vi "TableSandbox.vi"() -> ()   [LabVIEW 2013]
uses:
  <vilib>/Utility/miscctls.llb/LVRowAndColumnTypeDef.ctl
  <vilib>/Utility/miscctls.llb/LVBoundsTypeDef.ctl
  <vilib>/Utility/miscctls.llb/LVFontTypeDef.ctl
  <vilib>/Utility/miscctls.llb/LVPositionTypeDef.ctl
  <vilib>/Utility/miscctls.llb/LVRowAndColumnUnsignedTypeDef.ctl
  <vilib>/event_ctls.llb/eventsource.ctl
  <vilib>/event_ctls.llb/lveventtype.ctl
  <vilib>/Utility/miscctls.llb/LVPoint32TypeDef.ctl
  <vilib>/event_ctls.llb/eventvkey.ctl
  <vilib>/Utility/cursorutil.llb/Set Cursor (Icon Pict).vi
panel:
  out "Mouse\nUp":bool
  out "Mouse\nDown":bool
  out "data cols":i32
  out "data rows":i32
  in  "Enable diagnostics?":bool
  out "Active Cell:Cell Size":T1
  out "Color Box 3":u32(colorbox)
  out "Invoke: Point to Row-Column":cluster{"Cell Position":T2, "In Bounds?":bool}
  out "Active Cell:Position":T3
  out "Color Box 2":u32(colorbox)
  out "Active Cell:Cell Justification":enum16{"Left", "Center", "Right"}(ring)
  out "Active Cell:Cell Font":T4
  out "Active Cell:Cell Background Color":u32
  out "Active Cell:Active Cell":T2
  out "Row Header \nStrings[]":string[](array[string])
  out "Number of Rows":u32
  out "Number of Columns":u32
  out "Index Values":T5
  out "Edit Position":T2
  out "Content Rect\nPosition":T3
  out "Content Rect\nBounds":T1
  out "Size":T1
  out "Column Header \nStrings[]":string[](array[string])
  out "Autosizing Row Height":bool
  out "Visible Items:Vertical Scrollbar Visible":bool
  out "Visible Items:Vertical Lines Visible":bool
  out "Visible Items:Row Headers Visible":bool
  out "Visible Items:Index Visible":bool
  out "Visible Items:Horizontal Scrollbar Visible":bool
  out "Visible Items:Horizontal Lines Visible":bool
  out "Visible Items:Column Headers Visible":bool
  out "Smooth Horizontal Scrolling":bool
  out "Color Box":u32(colorbox)
  out "Selection Start":T2
  out "Selection Size":T2
  out "Selection Color":u32
  in  "Mode Col":i32=5
  in  "Tab Control":enum32{"Mouse Events", "Keyboard events"}(tab)
  out "Mouse Move\nIn Bounds?":bool
  out "Mouse Move\nCell Position":T2
  out "Mouse Move":T9={"Source"=0, "Type"=enum."Value Change", "Time"=0, "CtlRef"=refnum, "Coords"={"Horizontal"=0, "Vertical"=0}} {"Source" items=["LabVIEW UI"=0, "ActiveX"=1, "User Event"=25]}
  out "Mouse Leave":T10={"Source"=0, "Type"=enum."Value Change", "Time"=0, "CtlRef"=refnum} {"Source" items=["LabVIEW UI"=0, "ActiveX"=1, "User Event"=25]}
  out "Mouse Enter":T10={"Source"=0, "Type"=enum."Value Change", "Time"=0, "CtlRef"=refnum} {"Source" items=["LabVIEW UI"=0, "ActiveX"=1, "User Event"=25]}
  out "Mouse Up Event":T11={"Source"=0, "Type"=enum."Value Change", "Time"=0, "CtlRef"=refnum, "Coords"={"Horizontal"=0, "Vertical"=0}, "Button"=0, "Mods"={"Double Click"=FALSE, "Menu Key"=FALSE}, "PlatMods"={"Shift"=FALSE, "Ctrl"=FALSE, "Alt"=FALSE, "Cmd"=FALSE, "Opt"=FALSE}, "Invoke: Coords to row-col"={"In Bounds?"=FALSE, "Cell Position"={"Row"=0, "Column"=0}}} {"Source" items=["LabVIEW UI"=0, "ActiveX"=1, "User Event"=25]}
  out "down within digitals?":bool
  out "Shortcut Menu Activation? Event":T12={"Source"=0, "Type"=enum."Value Change", "Time"=0, "CtlRef"=refnum, "MenuRef"=refnum, "Coords"={"Horizontal"=0, "Vertical"=0}, "SubObj"=refnum, "Invoke: Coords to row-col"={"In Bounds?"=FALSE, "Cell Position"={"Row"=0, "Column"=0}}} {"Source" items=["LabVIEW UI"=0, "ActiveX"=1, "User Event"=25]}
  out "Mouse Down Event":T11={"Source"=0, "Type"=enum."Value Change", "Time"=0, "CtlRef"=refnum, "Coords"={"Horizontal"=0, "Vertical"=0}, "Button"=0, "Mods"={"Double Click"=FALSE, "Menu Key"=FALSE}, "PlatMods"={"Shift"=FALSE, "Ctrl"=FALSE, "Alt"=FALSE, "Cmd"=FALSE, "Opt"=FALSE}, "Invoke: Coords to row-col"={"In Bounds?"=FALSE, "Cell Position"={"Row"=0, "Column"=0}}} {"Source" items=["LabVIEW UI"=0, "ActiveX"=1, "User Event"=25]}
  out "down within edit":bool
  out "Button \n(Mouse Down?)":u16
  out "Key Down Event":T14={"Source"=0, "Type"=enum."Value Change", "Time"=0, "CtlRef"=refnum, "Char"=0, "VKey"=enum."ASCII", "ScanCode"=0, "Mods"={"Num Pad"=FALSE, "Menu Key"=FALSE}, "PlatMods"={"Shift"=FALSE, "Ctrl"=FALSE, "Alt"=FALSE, "Cmd"=FALSE, "Opt"=FALSE}, "FocusObj"=refnum} {"Source" items=["LabVIEW UI"=0, "ActiveX"=1, "User Event"=25]}
  out "Edit Position\n(loop st)":T2
  out "Edit Position\n(loop end)":T2
  out "Edit Position (down)":T2
  in  "Change \ncursor?":bool
  out "Mouse Down\nPosition":T2
  in  "Digital cols":i32=5
  in  "Digital rows":i32=5
  in  "Set Active Cell:\nActive Cell":T2
  in  "stop":bool
  in  "Table Control":string[][](table)
  # "Initialize"
  # "- toggle on dbl click\n- hold-click + type\n- Check if edit position exists and then \ncheck if same after click!"
  # "Diagnostics: Read all Property Node properties"
  # "Programmatic Control"
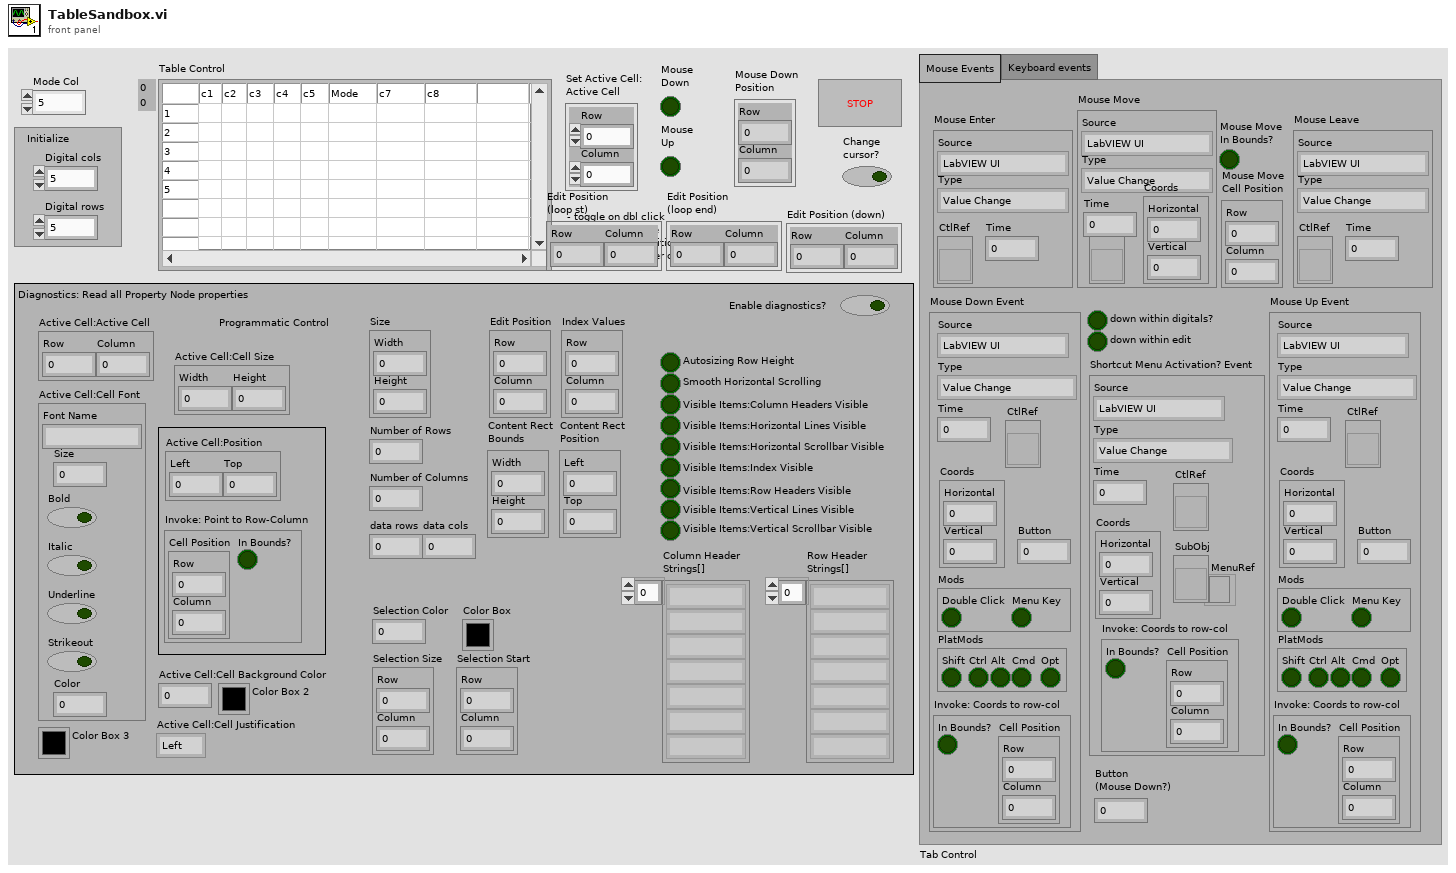
[diagram p1: front panel]
types:
  T1 = typedef "LVBoundsTypeDef.ctl" = cluster{"Width":u32, "Height":u32}
  T2 = typedef "LVRowAndColumnTypeDef.ctl" = cluster{"Row":i32, "Column":i32}
  T3 = typedef "LVPositionTypeDef.ctl" = cluster{"Left":i32, "Top":i32}
  T4 = typedef "LVFontTypeDef.ctl" = cluster{"Font Name":string, "Size":u16, "Bold":bool, "Italic":bool, "Underline":bool, "Strikeout":bool, "Color":u32}
  T5 = typedef "LVRowAndColumnUnsignedTypeDef.ctl" = cluster{"Row":u32, "Column":u32}
  T6 = typedef "eventsource.ctl" = u32
  T7 = typedef "lveventtype.ctl" = enum32{"Null", "Timeout", "Annotation Menu Selection", "Annotation Menu Selection?", "App Instance Close", "App Instance Close?", "Autoscale Range Change", "Bookmark Info Change", "Cell Edit", "Cell Edit?", "Cursor Grab", "Cursor Grab?", "Cursor Menu Selection", "Cursor Menu Selection?", "Cursor Move", "Cursor Release", "Data Change", "Direction Change", "Display State Change", "Drag Ended", "Drag Enter", "Drag Leave", "Drag Over", "Drag Source Update", "Drag Starting", "Drag Starting?", "Drop", "Exec State Change", "Key Down", "Key Down?", "Key Repeat", "Key Repeat?", "Key Up", "Listbox Double Click", "Menu Activation?", "Menu Selection (App)", "Menu Selection? (App)", "Menu Selection (User)", "Mouse Down", "Mouse Down?", "Mouse Enter", "Mouse Leave", "Mouse Move", "Mouse Up", "Mouse Wheel", "NI Security User Change (App)", "Pane Size", "Panel Close", "Panel Close?", "Panel Resize", "Plot Attribute Change", "Scale Range Change", "Shortcut Menu Activation?", "Shortcut Menu Selection (App)", "Shortcut Menu Selection? (App)", "Shortcut Menu Selection (User)", "Tree Double Click", "Tree Drag", "Tree Drag?", "Tree Drop", "Tree Drop?", "Tree Item Close", "Tree Item Close?", "Tree Item Open", "Tree Item Open?", "User Event", "Value Change"}
  T8 = typedef "LVPoint32TypeDef.ctl" = cluster{"Horizontal":i32, "Vertical":i32}
  T9 = cluster{"Source":T6, "Type":T7, "Time":u32, "CtlRef":refnum<vi>, "Coords":T8}
  T10 = cluster{"Source":T6, "Type":T7, "Time":u32, "CtlRef":refnum<vi>}
  T11 = cluster{"Source":T6, "Type":T7, "Time":u32, "CtlRef":refnum<vi>, "Coords":T8, "Button":u16, "Mods":cluster{"Double Click":bool, "Menu Key":bool}, "PlatMods":cluster{"Shift":bool, "Ctrl":bool, "Alt":bool, "Cmd":bool, "Opt":bool}, "Invoke: Coords to row-col":cluster{"In Bounds?":bool, "Cell Position":T2}}
  T12 = cluster{"Source":T6, "Type":T7, "Time":u32, "CtlRef":refnum<vi>, "MenuRef":refnum<k9>, "Coords":T8, "SubObj":refnum<vi>, "Invoke: Coords to row-col":cluster{"In Bounds?":bool, "Cell Position":T2}}
  T13 = typedef "eventvkey.ctl" = enum16{"ASCII", "Enter", "Return", "Shift", "Ctrl", "Alt", "Cmd", "Opt", "Caps", "NumLock", "Clear", "Break", "Up", "Down", "Left", "Right", "Insert", "Delete", "Home", "End", "PageUp", "PageDown", "Escape", "Help", "Pause", "ScrollLock", "F1", "F2", "F3", "F4", "F5", "F6", "F7", "F8", "F9", "F10", "F11", "F12", "F13", "F14", "F15", "F16", "F17", "F18", "F19", "F20", "F21", "F22", "F23", "F24", "Play", "VolumeUp", "VolumeDown", "Mute", "Two Byte Char"}
  T14 = cluster{"Source":T6, "Type":T7, "Time":u32, "CtlRef":refnum<vi>, "Char":i16, "VKey":T13, "ScanCode":i16, "Mods":cluster{"Num Pad":bool, "Menu Key":bool}, "PlatMods":cluster{"Shift":bool, "Ctrl":bool, "Alt":bool, "Cmd":bool, "Opt":bool}, "FocusObj":refnum<vi>}
  T15 = cluster{"Shift":bool, "Ctrl":bool, "Alt":bool, "Cmd":bool, "Opt":bool}
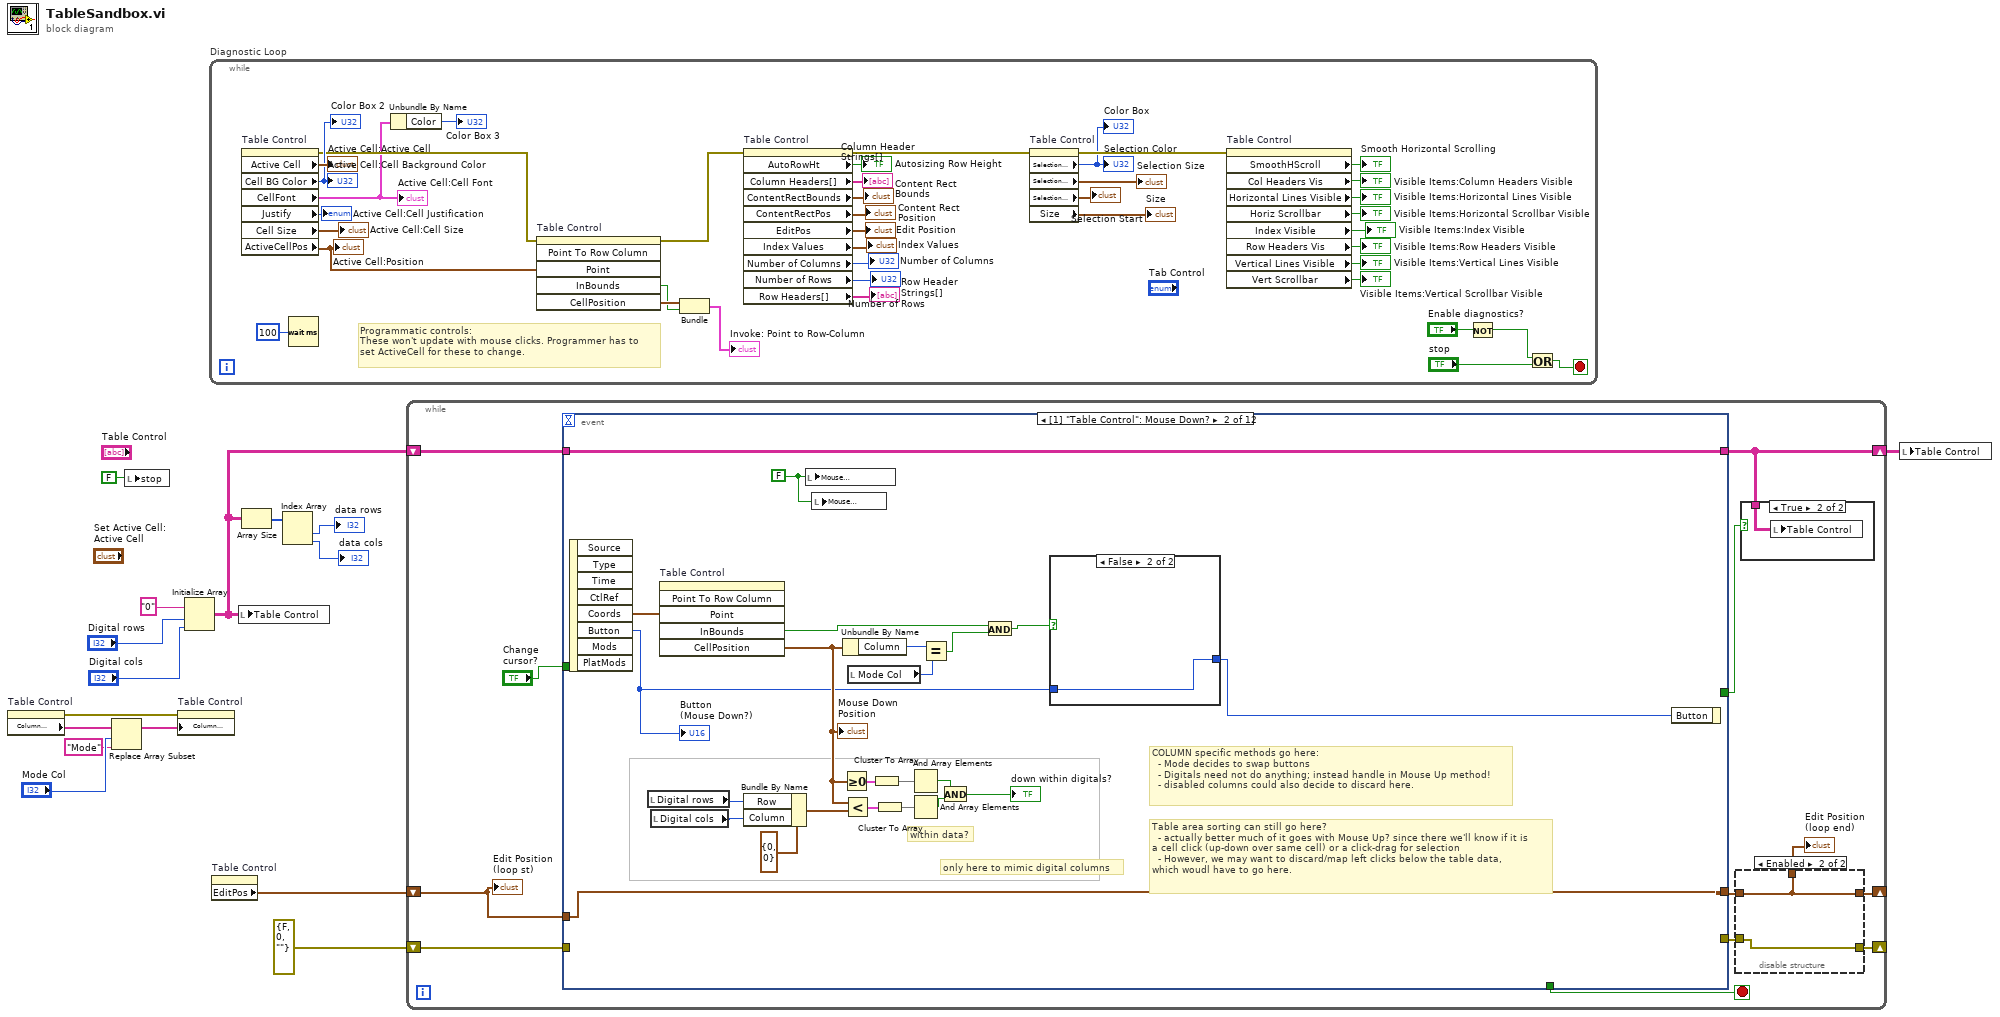
[diagram p0: block diagram]
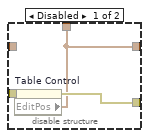
[diagram p2: hidden frame]
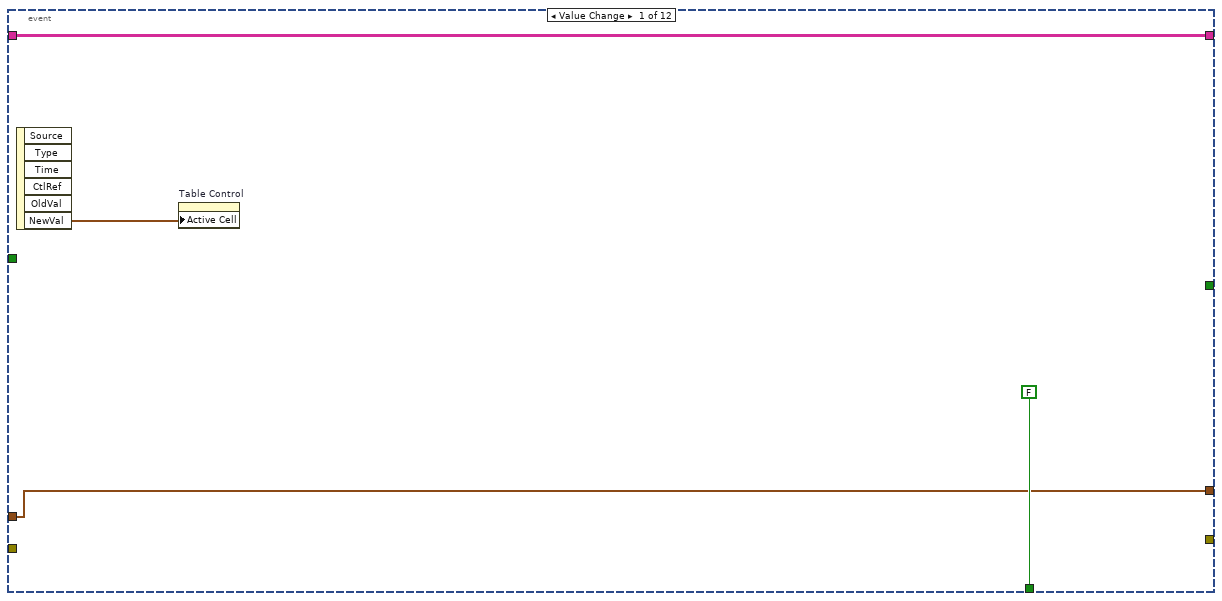
[diagram p4: hidden frame]
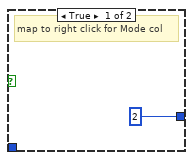
[diagram p5: hidden frame]
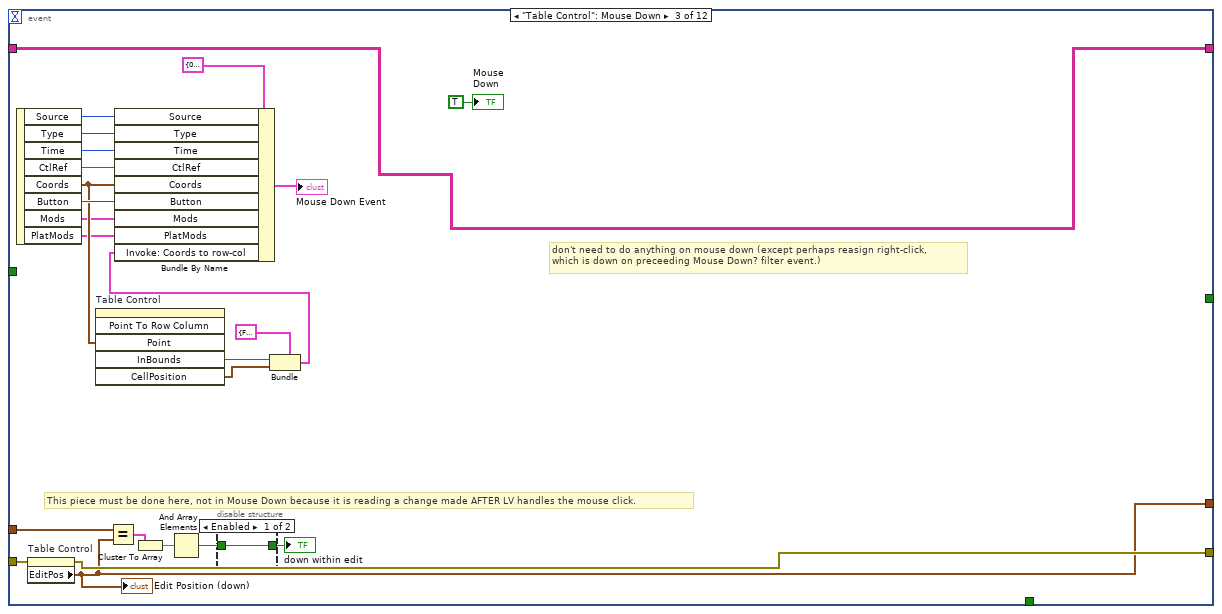
[diagram p6: hidden frame]
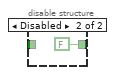
[diagram p7: hidden frame]
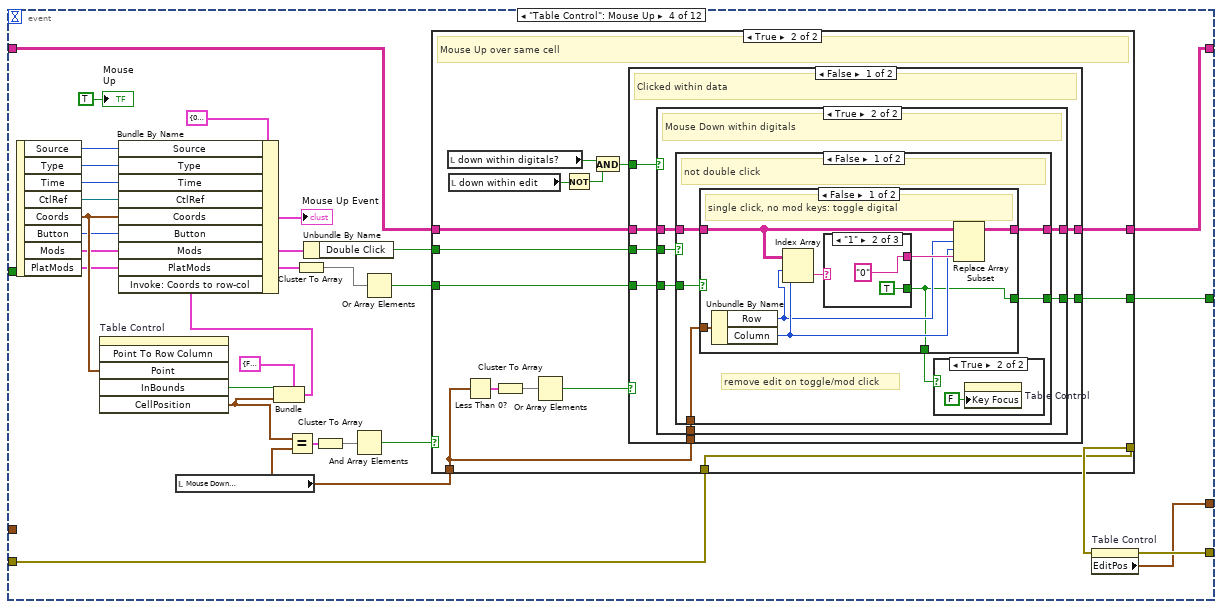
[diagram p8: hidden frame]
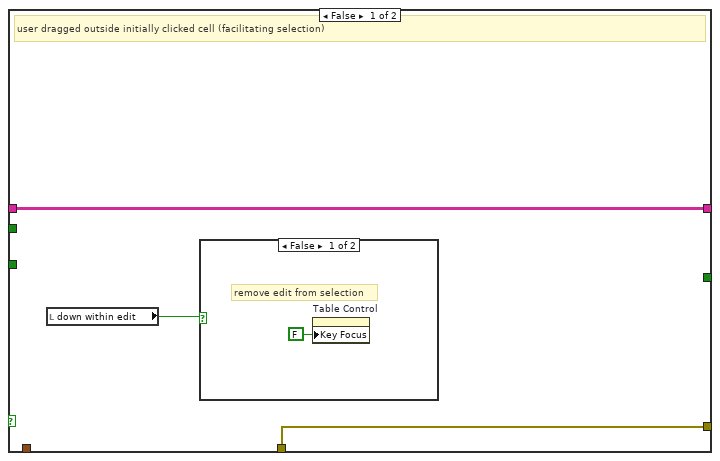
[diagram p9: hidden frame]
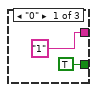
[diagram p13: hidden frame]
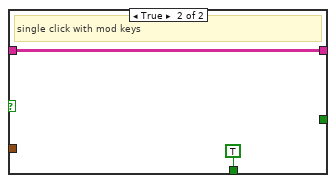
[diagram p15: hidden frame]
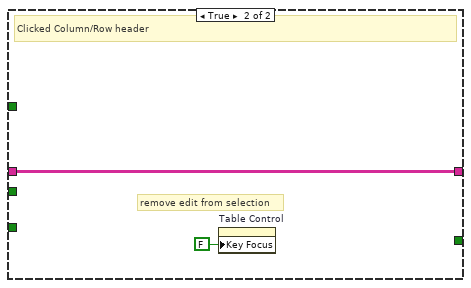
[diagram p17: hidden frame]
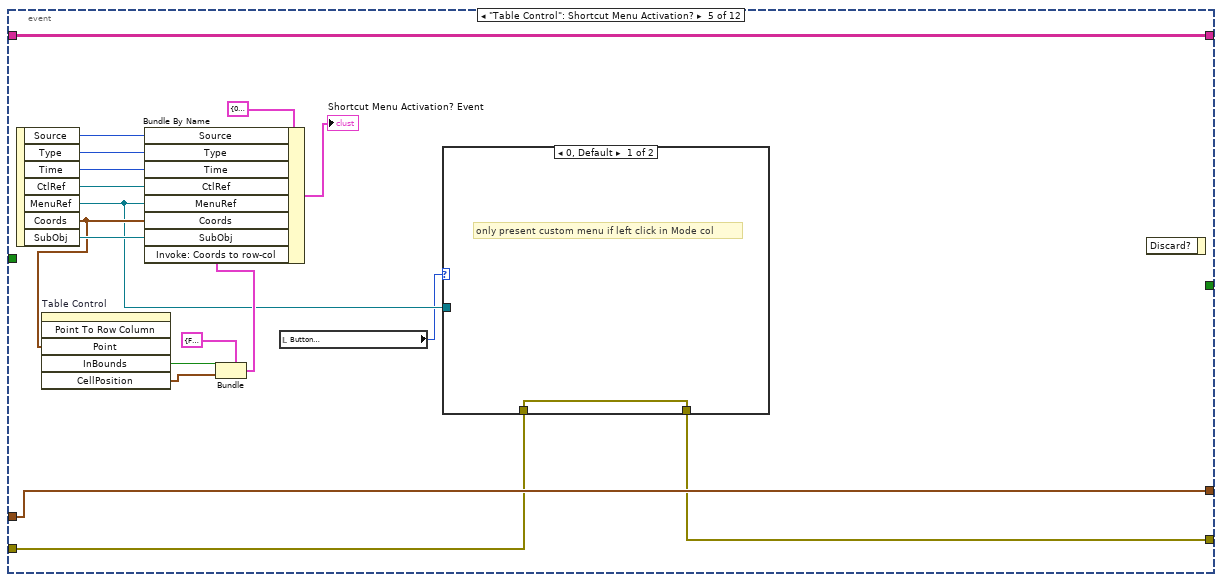
[diagram p18: hidden frame]
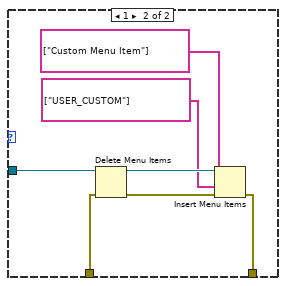
[diagram p19: hidden frame]
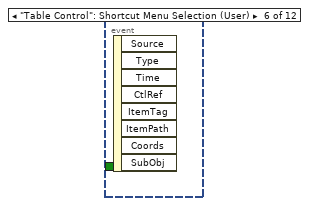
[diagram p20: hidden frame]
diagram:
  n1 = property on="Table Control" class="Tbl (strict)"() -> (error out=w6:errorcluster, "Column Headers[]"=w9:string[])  [unwired: 2 in, 1 out]
  n2 = Replace Array Subset(array=w9, new element="Mode" ("new element/subarray"), index="Mode Col") -> (w5:string[])
  n3 = local write "stop"(FALSE ("stop")) -> ()
  n4 = property on="Table Control" class="Tbl (strict)"(error in=w6, "Column Headers[]"=w5) -> ()  [unwired: 1 in, 2 out]
  n5 = Initialize Array("0", "Digital rows", "Digital cols") -> (w4:string[][])
  n6 = while "Diagnostic Loop" {
    stop <- w19 stop-if-true
    # "Programmatic controls:\nThese won't update with mouse clicks. Programmer has to\nset ActiveCell for these to change."
    n7 = property on="Table Control" class="Tbl (strict)"() -> (error out=w37:errorcluster, "Active Cell"=→"Active Cell:Active Cell":T2, "Cell BG Color"=→"Active Cell:Cell Background Color" →"Color Box 2":u32, "CellFont"=w35:T4, "Justify"=→"Active Cell:Cell Justification":enum16{"Left", "Center", "Right"}, "Cell Size"=→"Active Cell:Cell Size":T1, "ActiveCellPos"=w38:T3)  [unwired: 2 in, 1 out]
    "Active Cell:Cell Font" <- w35
    "Active Cell:Position" <- w38
    n8 = Wait (ms)(milliseconds to wait=u32 100) -> ()  [unwired: 1 out]
    n9 = Unbundle By Name(w35) -> ("Color"=→"Color Box 3":u32)
    n10 = invoke on="Table Control" class="Tbl (strict)" method="Point To Row Column"(error in=w37, "Point"=w38) -> (error out=w36:errorcluster, "InBounds"=w32:bool, "CellPosition"=w33:T2)  [unwired: 4 in, 3 out]
    n11 = Bundle("CellPosition"=w33, "InBounds"=w32) -> (→"Invoke: Point to Row-Column":cluster{"CellPosition":T2, "InBounds":bool})  [unwired: 1 in]
    n12 = property on="Table Control" class="Tbl (strict)"(error in=w36) -> (error out=w55:errorcluster, "AutoRowHt"=→"Autosizing Row Height":bool, "Column Headers[]"=→"Column Header \nStrings[]":string[], "ContentRectBounds"=→"Content Rect\nBounds":T1, "ContentRectPos"=→"Content Rect\nPosition":T3, "EditPos"=→"Edit Position":T2, "Index Values"=→"Index Values":T5, "Number of Columns"=→"Number of Columns":u32, "Number of Rows"=→"Number of Rows":u32, "Row Headers[]"=→"Row Header \nStrings[]":string[])  [unwired: 1 in, 1 out]
    n13 = property on="Table Control" class="Tbl (strict)"(error in=w55) -> (error out=w56:errorcluster, "Selection Color"=→"Selection Color" →"Color Box":u32, "Selection Size"=→"Selection Size":T2, "Selection Start"=→"Selection Start":T2, "Size"=→"Size":T1)  [unwired: 1 in, 1 out]
    n14 = property on="Table Control" class="Tbl (strict)"(error in=w56) -> ("SmoothHScroll"=→"Smooth Horizontal Scrolling":bool, "Col Headers Vis"=→"Visible Items:Column Headers Visible":bool, "Horizontal Lines Visible"=→"Visible Items:Horizontal Lines Visible":bool, "Horiz Scrollbar"=→"Visible Items:Horizontal Scrollbar Visible":bool, "Index Visible"=→"Visible Items:Index Visible":bool, "Row Headers Vis"=→"Visible Items:Row Headers Visible":bool, "Vertical Lines Visible"=→"Visible Items:Vertical Lines Visible":bool, "Vert Scrollbar"=→"Visible Items:Vertical Scrollbar Visible":bool)  [unwired: 1 in, 2 out]
    n15 = Not(x="Enable diagnostics?") -> (.not. x?=w17:bool)
    n16 = Or(x=w17, y="stop") -> (x .or. y?=w19:bool)
  }
  n17 = property on="Table Control" class="Tbl (strict)"() -> ("EditPos"=w10:T2)  [unwired: 2 in, 2 out]
  n18 = local write "Table Control"(w4) -> ()
  n19 = Array Size(array=w4) -> (size(s)=w3:i32[])
  n20 = Index Array(array=w3) -> (element #1=→"data rows":i32, element #2=→"data cols":i32)  [unwired: 2 in]
  n21 = while {
    shift-right: [w66] -> w12
    shift-left: w4 -> [w67]
    shift-right: [w61] -> _
    shift-left: errorcluster {"status"=FALSE, "code"=0, "source"=""} ("error in (no error)") -> [w62]
    shift-right: [w60] -> _
    shift-left: w10 -> [w59]
    stop <- w68 stop-if-true
    n22 = event shown="[1] \"Table Control\": Mouse Down?" {
      selector: _ -> [_ _ _ _ _ _ _ _ _ _ _ _]
      dyn-events: _ -> [_ _ _ _ _ _ _ _ _ _ _ _]
      timeout: _ -> [_ _ _ _ _ _ _ _ _ _ _ _]
      tunnel: [FALSE _ _ _ _ _ _ _ _ _ _ TRUE] -> w68
      tunnel: w67 -> [w76 w101 w115 w146 w221 _ _ w276 w296 w308 w330 w340]
      tunnel: [w76 w101 w115 w145 w221 _ w244 w276 w296 w308 w330 w340] -> w66
      tunnel: [_ _ _ w140 _ _ TRUE _ _ _ _ _] -> w65
      tunnel: "Change \ncursor?" -> [_ _ _ _ _ _ _ _ _ w305 w329 _]
      tunnel: [_ _ w112 w139 w218 _ w247 w251 _ _ _ _] -> w63
      tunnel: w62 -> [_ _ w111 w137 w219 _ w247 w263 _ _ _ _]
      tunnel: w59 -> [w75 w100 w110 _ w220 _ w246 _ w295 w303 w328 w339]
      tunnel: [w75 w100 w105 w138 w220 _ w246 w249 w295 w303 w328 w339] -> w58
      event Value Change {
        n23 = event-data() -> ("NewVal"=w78:T2)  [unwired: 1 in, 5 out]
        n24 = property on="Table Control" class="Tbl (strict)"("Active Cell"=w78) -> ()  [unwired: 2 in, 2 out]
      }
      event "Table Control": Mouse Down? {
        w80 = FALSE ("Mouse\nDown")
        # "Table area sorting can still go here?\n  - actually better much of it goes with Mouse Up? since there we'll know if it is\na cell click (up-down over same cell) or a click-drag for selection\n  - However, we may want to discard/map left clicks below the table data, \nwhich woudl have to go here."
        # "only here to mimic digital columns"
        # "COLUMN specific methods go here:\n  - Mode decides to swap buttons\n  - Digitals need not do anything; instead handle in Mouse Up method!\n  - disabled columns could also decide to discard here."
        # "within data?"
        n25 = event-data() -> ("Coords"=w99:T8, "Button"=w79:u16)  [unwired: 1 in, 6 out]
        "Button \n(Mouse Down?)" <- w79
        n26 = local read "Digital rows"() -> (w91:i32)
        n27 = local read "Digital cols"() -> (w90:i32)
        n28 = invoke on="Table Control" class="Tbl (strict)" method="Point To Row Column"("Point"=w99) -> ("InBounds"=w95:bool, "CellPosition"=w81:T2)  [unwired: 5 in, 4 out]
        "Mouse Down\nPosition" <- w81
        n29 = Bundle By Name(cluster=T2 {"Row"=0, "Column"=0} ("Cell Position"), "Row"=w91, "Column"=w90) -> (w89:T2)
        n30 = local write "Mouse\nDown"(w80) -> ()
        n31 = local write "Mouse\nUp"(w80) -> ()
        n32 = Greater Or Equal To 0?(x=w81) -> (x >= 0?=w83:cluster{"Row":bool, "Column":bool})
        n33 = Unbundle By Name(w81) -> ("Column"=w98:i32)
        n34 = Less?(x=w81, y=w89) -> (x < y?=w88:cluster{"Row":bool, "Column":bool})
        n35 = local read "Mode Col"() -> (w97:i32)
        n36 = Cluster To Array(cluster=w83) -> (array=w82:bool[])
        n37 = Cluster To Array(cluster=w88) -> (array=w87:bool[])
        n38 = And Array Elements(Boolean array=w82) -> (logical AND=w85:bool)
        n39 = And Array Elements(Boolean array=w87) -> (logical AND=w86:bool)
        n40 = Equal?(x=w98, y=w97) -> (x = y?=w96:bool)
        n41 = And(x=w85, y=w86) -> (x .and. y?=→"down within digitals?":bool)
        n42 = And(x=w95, y=w96) -> (x .and. y?=w94:bool)
        n43 = case shown="False" w94 {
          tunnel: [u16 2 ("Button") w103] -> w93
          tunnel: w79 -> [_ w103]
          frame True {
            # "map to right click for Mode col"
          }
          frame False {
          }
        }
        n44 = event-data("Button"=w93) -> ()  [unwired: 1 in, 1 out]
      }
      event "Table Control": Mouse Down {
        # "This piece must be done here, not in Mouse Down because it is reading a change made AFTER LV handles the mouse click."
        # "don't need to do anything on mouse down (except perhaps reasign right-click,\nwhich is down on preceeding Mouse Down? filter event.)"
        n45 = event-data() -> ("Source"=w127:T6, "Type"=w126:T7, "Time"=w125:u32, "CtlRef"=w124:refnum<vi>, "Coords"=w118:T8, "Button"=w123:u16, "Mods"=w114:cluster{"Double Click":bool, "Menu Key":bool}, "PlatMods"=w113:T15)  [unwired: 1 in]
        n46 = property on="Table Control" class="Tbl (strict)"(error in=w111) -> (error out=w112:errorcluster, "EditPos"=w105:T2)  [unwired: 1 in, 1 out]
        "Edit Position (down)" <- w105
        n47 = invoke on="Table Control" class="Tbl (strict)" method="Point To Row Column"("Point"=w118) -> ("InBounds"=w119:bool, "CellPosition"=w116:T2)  [unwired: 5 in, 4 out]
        n48 = Equal?(x=w110, y=w105) -> (x = y?=w109:cluster{"Row":bool, "Column":bool})
        n49 = Cluster To Array(cluster=w109) -> (array=w108:bool[])
        n50 = And Array Elements(Boolean array=w108) -> (logical AND=w107:bool)
        n51 = disable-structure shown="Enabled" {
          disable-tunnel: w107 -> [w128 _]
          disable-tunnel: [w128 FALSE ("down within edit")] -> w106
          frame Enabled {
          }
          frame Disabled {
          }
        }
        "down within edit" <- w106
        n52 = Bundle(cluster=cluster{"In Bounds?":bool, "Cell Position":T2} {"In Bounds?"=FALSE, "Cell Position"={"Row"=0, "Column"=0}} ("Invoke: Coords to row-col"), "In Bounds?"=w119, "Cell Position"=w116) -> (w117:cluster{"In Bounds?":bool, "Cell Position":T2})
        n53 = Bundle By Name(cluster=T11 {"Source"=0, "Type"=enum."Mouse Down", "Time"=108372288, "CtlRef"=refnum, "Coords"={"Horizontal"=318, "Vertical"=90}, "Button"=1, "Mods"={"Double Click"=FALSE, "Menu Key"=FALSE}, "PlatMods"={"Shift"=FALSE, "Ctrl"=FALSE, "Alt"=FALSE, "Cmd"=FALSE, "Opt"=FALSE}, "Invoke: Coords to row-col"={"In Bounds?"=TRUE, "Cell Position"={"Row"=0, "Column"=2}}} ("Mouse Down Event"), "Source"=w127, "Type"=w126, "Time"=w125, "CtlRef"=w124, "Coords"=w118, "Button"=w123, "Mods"=w114, "PlatMods"=w113, "Invoke: Coords to row-col"=w117) -> (→"Mouse Down Event":T11)
        "Mouse\nDown" <- TRUE ("Mouse\nDown")
      }
      event "Table Control": Mouse Up {
        n54 = event-data() -> ("Source"=w156:T6, "Type"=w155:T7, "Time"=w154:u32, "CtlRef"=w153:refnum<vi>, "Coords"=w152:T8, "Button"=w151:u16, "Mods"=w147:cluster{"Double Click":bool, "Menu Key":bool}, "PlatMods"=w143:T15)  [unwired: 1 in]
        n55 = invoke on="Table Control" class="Tbl (strict)" method="Point To Row Column"("Point"=w152) -> ("InBounds"=w150:bool, "CellPosition"=w133:T2)  [unwired: 5 in, 4 out]
        n56 = local read "Mouse Down\nPosition"() -> (w131:T2)
        n57 = Bundle(cluster=cluster{"In Bounds?":bool, "Cell Position":T2} {"In Bounds?"=FALSE, "Cell Position"={"Row"=0, "Column"=0}} ("Invoke: Coords to row-col"), "In Bounds?"=w150, "Cell Position"=w133) -> (w149:cluster{"In Bounds?":bool, "Cell Position":T2})
        n58 = Bundle By Name(cluster=T11 {"Source"=0, "Type"=enum."Mouse Down", "Time"=108372288, "CtlRef"=refnum, "Coords"={"Horizontal"=318, "Vertical"=90}, "Button"=1, "Mods"={"Double Click"=FALSE, "Menu Key"=FALSE}, "PlatMods"={"Shift"=FALSE, "Ctrl"=FALSE, "Alt"=FALSE, "Cmd"=FALSE, "Opt"=FALSE}, "Invoke: Coords to row-col"={"In Bounds?"=TRUE, "Cell Position"={"Row"=0, "Column"=2}}} ("Mouse Down Event"), "Source"=w156, "Type"=w155, "Time"=w154, "CtlRef"=w153, "Coords"=w152, "Button"=w151, "Mods"=w147, "PlatMods"=w143, "Invoke: Coords to row-col"=w149) -> (→"Mouse Up Event":T11)
        n59 = Equal?(x=w133, y=w131) -> (x = y?=w134:cluster{"Row":bool, "Column":bool})
        n60 = Cluster To Array(cluster=w143) -> (array=w142:bool[])
        n61 = Unbundle By Name(w147) -> ("Double Click"=w144:bool)
        n62 = Cluster To Array(cluster=w134) -> (array=w135:bool[])
        n63 = And Array Elements(Boolean array=w135) -> (logical AND=w132:bool)
        n64 = Or Array Elements(Boolean array=w142) -> (logical OR=w141:bool)
        n65 = case shown="True" w132 {
          tunnel: w146 -> [w161 w176]
          tunnel: [w161 w175] -> w145
          tunnel: w144 -> [_ w167]
          tunnel: w141 -> [_ w174]
          tunnel: [_ w173] -> w140
          tunnel: w137 -> [w160 w172]
          tunnel: [w160 w172] -> w136
          tunnel: w131 -> [_ w166]
          frame False {
            # "user dragged outside initially clicked cell (facilitating selection)"
            n66 = local read "down within edit"() -> (w159:bool)
            n67 = case shown="False" w159 {
              frame False {
                # "remove edit from selection"
                n68 = property on="Table Control" class="Tbl (strict)"("Key Focus"=FALSE) -> ()  [unwired: 2 in, 2 out]
              }
              frame True {
              }
            }
          }
          frame True {
            # "Mouse Up over same cell"
            n69 = local read "down within digitals?"() -> (w170:bool)
            n70 = local read "down within edit"() -> (w169:bool)
            n71 = Less Than 0?(x=w166) -> (x < 0?=w165:cluster{"Row":bool, "Column":bool})
            n72 = Cluster To Array(cluster=w165) -> (array=w164:bool[])
            n73 = Or Array Elements(Boolean array=w164) -> (logical OR=w163:bool)
            n74 = Not(x=w169) -> (.not. x?=w171:bool)
            n75 = And(x=w170, y=w171) -> (x .and. y?=w168:bool)
            n76 = case shown="False" w163 {
              tunnel: w176 -> [w183 w214]
              tunnel: [w182 w214] -> w175
              tunnel: w174 -> [w181 _]
              tunnel: [w180 _] -> w173
              tunnel: w168 -> [w179 _]
              tunnel: w167 -> [w178 _]
              tunnel: w166 -> [w177 _]
              frame False {
                # "Clicked within data"
                n77 = case shown="True" w179 {
                  tunnel: w183 -> [w184 w190]
                  tunnel: [w184 w189] -> w182
                  tunnel: w178 -> [_ w188]
                  tunnel: w181 -> [_ w187]
                  tunnel: [_ w186] -> w180
                  tunnel: w177 -> [_ w185]
                  frame False {
                    # "Mouse down in non-digital cell (let LV handle entirely)"
                  }
                  frame True {
                    # "Mouse Down within digitals"
                    n78 = case shown="False" w188 {
                      tunnel: w190 -> [w196 w213]
                      tunnel: [w195 w213] -> w189
                      tunnel: w187 -> [w194 _]
                      tunnel: [w193 _] -> w186
                      tunnel: w185 -> [w191 _]
                      frame False {
                        # "remove edit on toggle/mod click"
                        # "not double click"
                        n79 = case shown="False" w194 {
                          tunnel: w196 -> [w203 w212]
                          tunnel: [w200 w212] -> w195
                          tunnel: [w199 _] -> w193
                          tunnel: [w199 TRUE] -> w192
                          tunnel: w191 -> [w198 _]
                          frame False {
                            # "single click, no mod keys: toggle digital"
                            n80 = Unbundle By Name(w198) -> ("Row"=w201:i32, "Column"=w202:i32)
                            n81 = Index Array(array=w203, index (row)=w201, index (col)=w202) -> (element=w205:string)
                            n82 = case shown="\"1\"" w205 {
                              selector: w205 -> [_ _ w210]
                              tunnel: ["1" "0" w210] -> w204
                              tunnel: [TRUE TRUE _] -> w199
                              frame "0" {
                              }
                              frame "1" {
                              }
                              frame Default {
                              }
                            }
                            n83 = Replace Array Subset(array=w203, new element=w204, index (row)=w201, index (col)=w202) -> (w200:string[][])
                          }
                          frame True {
                            # "single click with mod keys"
                          }
                        }
                        n84 = case shown="True" w192 {
                          frame False {
                          }
                          frame True {
                            n85 = property on="Table Control" class="Tbl (strict)"("Key Focus"=FALSE) -> ()  [unwired: 2 in, 2 out]
                          }
                        }
                      }
                      frame True {
                        # "double click: do nothing (bring up edit)"
                      }
                    }
                  }
                }
              }
              frame True {
                # "remove edit from selection"
                # "Clicked Column/Row header"
                n86 = property on="Table Control" class="Tbl (strict)"("Key Focus"=FALSE) -> ()  [unwired: 2 in, 2 out]
              }
            }
          }
        }
        n87 = property on="Table Control" class="Tbl (strict)"(error in=w136) -> (error out=w139:errorcluster, "EditPos"=w138:T2)  [unwired: 1 in, 1 out]
        "Mouse\nUp" <- TRUE ("Mouse\nUp")
      }
      event "Table Control": Shortcut Menu Activation? {
        n88 = event-data() -> ("Source"=w233:T6, "Type"=w232:T7, "Time"=w231:u32, "CtlRef"=w230:refnum<vi>, "MenuRef"=w217:refnum<k9>, "Coords"=w228:T8, "SubObj"=w229:refnum<vi>)  [unwired: 1 in]
        n89 = invoke on="Table Control" class="Tbl (strict)" method="Point To Row Column"("Point"=w228) -> ("InBounds"=w225:bool, "CellPosition"=w222:T2)  [unwired: 5 in, 4 out]
        n90 = Bundle(cluster=cluster{"In Bounds?":bool, "Cell Position":T2} {"In Bounds?"=FALSE, "Cell Position"={"Row"=0, "Column"=0}} ("Invoke: Coords to row-col"), "In Bounds?"=w225, "Cell Position"=w222) -> (w224:cluster{"In Bounds?":bool, "Cell Position":T2})
        n91 = Bundle By Name(cluster=T12 {"Source"=0, "Type"=enum."Value Change", "Time"=0, "CtlRef"=refnum, "MenuRef"=refnum, "Coords"={"Horizontal"=0, "Vertical"=0}, "SubObj"=refnum, "Invoke: Coords to row-col"={"In Bounds?"=TRUE, "Cell Position"={"Row"=0, "Column"=2}}} ("Shortcut Menu Activation? Event"), "Source"=w233, "Type"=w232, "Time"=w231, "CtlRef"=w230, "MenuRef"=w217, "Coords"=w228, "SubObj"=w229, "Invoke: Coords to row-col"=w224) -> (→"Shortcut Menu Activation? Event":T12)
        n92 = local read "Button \n(Mouse Down?)"() -> (w216:u16)
        n93 = case shown="0, Default" w216 {
          tunnel: w219 -> [w234 w240]
          tunnel: [w234 w239] -> w218
          tunnel: w217 -> [_ w238]
          frame 0, Default {
            # "only present custom menu if left click in Mode col"
          }
          frame 1 {
            n94 = Delete Menu Items(6:w240, 9:w238) -> (0:w241:errorcluster, 3:w237:refnum<k9>)  [unwired: 2 in]
            n95 = Insert Menu Items(6:w241, 7:string[] ["USER_CUSTOM"] ("item names"), 8:string[] ["Custom Menu Item"] ("item names"), 9:w237) -> (0:w239:errorcluster)  [unwired: 2 in, 2 out]
          }
        }
        n96 = event-data() -> ()  [unwired: 2 in, 1 out]
      }
      event "Table Control": Shortcut Menu Selection (User) {
        n97 = event-data() -> ()  [unwired: 1 in, 8 out]
      }
      event "Table Control": Value Change {
        # "must include this event since I have the data in the table as a shift register\non the event loop! Otherwise, the next event has an old version of the table \nand overwrites user edits."
        n98 = event-data() -> ("NewVal"=w244:string[][])  [unwired: 1 in, 5 out]
        n99 = Array Size(array=w244) -> (size(s)=w245:i32[])
        n100 = Index Array(array=w245) -> (element #1=w243:i32, element #2=w242:i32)  [unwired: 2 in]
        n101 = local write "data rows"(w243) -> ()
        n102 = local write "data cols"(w242) -> ()
      }
      event "Table Control": Key Down {
        # "This is imperfect: Shift-tab gets stuck when moving to the left.\nAlso, shift-arrows allow free keyboard navigation. Need to disallow header row navigation!\nWith so many cases to handle, may be best to add as subVI!"
        # "Handle keyboard navigation."
        # "Also need to handle if edit position is moved outside the data area."
        # "Even if we do nothing on Key Down, require event since\npressing tab or enter can change the Edit Positon. \nThus, the loop runs when event occurs and the edit positon is updated."
        n103 = event-data() -> ("Source"=w273:T6, "Type"=w272:T7, "Time"=w271:u32, "CtlRef"=w270:refnum<vi>, "Char"=w269:i16, "VKey"=w268:T13, "ScanCode"=w267:i16, "Mods"=w266:cluster{"Num Pad":bool, "Menu Key":bool}, "PlatMods"=w265:T15, "FocusObj"=w264:refnum<vi>)  [unwired: 1 in]
        n104 = Bundle By Name(cluster=T14 {"Source"=0, "Type"=enum."Value Change", "Time"=0, "CtlRef"=refnum, "Char"=0, "VKey"=enum."ASCII", "ScanCode"=0, "Mods"={"Num Pad"=FALSE, "Menu Key"=FALSE}, "PlatMods"={"Shift"=FALSE, "Ctrl"=FALSE, "Alt"=FALSE, "Cmd"=FALSE, "Opt"=FALSE}, "FocusObj"=refnum} ("Key Down Event"), "Source"=w273, "Type"=w272, "Time"=w271, "CtlRef"=w270, "Char"=w269, "VKey"=w268, "ScanCode"=w267, "Mods"=w266, "PlatMods"=w265, "FocusObj"=w264) -> (→"Key Down Event":T14)
        n105 = property on="Table Control" class="Tbl (strict)"(error in=w263) -> (error out=w260:errorcluster, "EditPos"=w258:T2)  [unwired: 1 in, 1 out]
        n106 = local read "data rows"() -> (w262:i32)
        n107 = Unbundle By Name(w258) -> ("Row"=w261:i32, "Column"=w257:i32)
        n108 = Greater?(x=w262, y=w261) -> (0:w259:bool)
        n109 = case shown="False" w259 {
          tunnel: w260 -> [w292 w294]
          tunnel: [w291 w294] -> w252
          tunnel: w258 -> [w290 w293]
          tunnel: [w289 w293] -> w250
          tunnel: w257 -> [w287 _]
          frame False {
            # "enter took edit below row bounds"
            n110 = Increment(x=w287) -> (x+1=w286:i32)
            n111 = Bundle By Name(cluster=w290, "Row"=0, "Column"=w286) -> (w289:T2)
            n112 = property on="Table Control" class="Tbl (strict)"(error in=w292, "EditPos"=w289) -> (error out=w291:errorcluster)  [unwired: 1 in, 1 out]
          }
          frame True {
          }
        }
        n113 = local read "data cols"() -> (w255:i32)
        n114 = Unbundle By Name(w250) -> ("Column"=w254:i32, "Row"=w256:i32)
        n115 = Greater?(x=w255, y=w254) -> (0:w253:bool)
        n116 = case shown="False" w253 {
          tunnel: w252 -> [w283 w285]
          tunnel: [w282 w285] -> w251
          tunnel: w250 -> [w281 w284]
          tunnel: [w280 w284] -> w249
          tunnel: w256 -> [w278 _]
          frame False {
            # "tab took edit past column bounds"
            n117 = Increment(x=w278) -> (x+1=w277:i32)
            n118 = Bundle By Name(cluster=w281, "Column"=0 ("Row"), "Row"=w277) -> (w280:T2)
            n119 = property on="Table Control" class="Tbl (strict)"(error in=w283, "EditPos"=w280) -> (error out=w282:errorcluster)  [unwired: 1 in, 1 out]
          }
          frame True {
          }
        }
      }
      event "Table Control": Mouse Enter {
        n120 = event-data() -> ("Source"=w301:T6, "Type"=w300:T7, "Time"=w299:u32, "CtlRef"=w298:refnum<vi>)  [unwired: 1 in]
        n121 = Bundle By Name(cluster=T10 {"Source"=0, "Type"=enum."Value Change", "Time"=0, "CtlRef"=refnum} ("Cluster 2"), "Source"=w301, "Type"=w300, "Time"=w299, "CtlRef"=w298) -> (→"Mouse Enter":T10)
      }
      event "Table Control": Mouse Move {
        n122 = event-data() -> ("Source"=w312:T6, "Type"=w311:T7, "Time"=w310:u32, "CtlRef"=w309:refnum<vi>, "Coords"=w307:T8)  [unwired: 1 in]
        n123 = disable-structure shown="Enabled" {
          disable-tunnel: w312 -> [w325 _]
          disable-tunnel: w311 -> [w324 _]
          disable-tunnel: w310 -> [w323 _]
          disable-tunnel: w309 -> [w322 _]
          disable-tunnel: w307 -> [w321 _]
          frame Enabled {
            n124 = Bundle By Name(cluster=T9 {"Source"=0, "Type"=enum."Value Change", "Time"=0, "CtlRef"=refnum, "Coords"={"Horizontal"=0, "Vertical"=0}} ("Mouse Move"), "Source"=w325, "Type"=w324, "Time"=w323, "CtlRef"=w322, "Coords"=w321) -> (→"Mouse Move":T9)
          }
          frame Disabled {
          }
        }
        n125 = invoke on="Table Control" class="Tbl (strict)" method="Point To Row Column"("Point"=w307) -> ("InBounds"=w304:bool, "CellPosition"=w306:T2)  [unwired: 5 in, 4 out]
        "Mouse Move\nCell Position" <- w306
        "Mouse Move\nIn Bounds?" <- w304
        n126 = case shown="True" w305 {
          tunnel: w306 -> [_ w318]
          tunnel: w304 -> [_ w314]
          frame False {
          }
          frame True {
            # "This code does not work!\nWhile the logic is OK, the actual cursor is only redrawn on a click?!"
            n127 = Greater Or Equal To 0?(x=w318) -> (x >= 0?=w317:cluster{"Row":bool, "Column":bool})
            n128 = Cluster To Array(cluster=w317) -> (array=w316:bool[])
            n129 = And Array Elements(Boolean array=w316) -> (logical AND=w313:bool)
            n130 = And(x=w314, y=w313) -> (x .and. y?=w315:bool)
            n131 = case shown="True" w315 {
              frame False {
                # "otherwise back to auto"
                n132 = call-poly <vilib>:"Set Cursor.vi"("icon"=u16 0) -> ()  [unwired: 9 in, 2 out]
              }
              frame True {
                # "set to hand over data\nbut not headers"
                n133 = call-poly <vilib>:"Set Cursor.vi"("icon"=u16 6) -> ()  [unwired: 9 in, 2 out]
              }
            }
          }
        }
      }
      event "Table Control": Mouse Leave {
        n134 = event-data() -> ("Source"=w335:T6, "Type"=w334:T7, "Time"=w333:u32, "CtlRef"=w332:refnum<vi>)  [unwired: 1 in]
        n135 = Bundle By Name(cluster=T10 {"Source"=0, "Type"=enum."Value Change", "Time"=0, "CtlRef"=refnum} ("Cluster 2"), "Source"=w335, "Type"=w334, "Time"=w333, "CtlRef"=w332) -> (→"Mouse Leave":T10)
        n136 = case shown="False" w329 {
          frame True {
            n137 = call-poly <vilib>:"Set Cursor.vi"("icon"=u16 0) -> ()  [unwired: 9 in, 2 out]
          }
          frame False {
            # "do nothing"
            n138 = disable-structure shown="Disabled" {
              frame Disabled {
                n139 = call-poly <vilib>:"Set Cursor.vi"("icon"=u16 0) -> ()  [unwired: 9 in, 2 out]
              }
              frame Enabled {
              }
            }
          }
        }
      }
      event "stop": Value Change {
        n140 = event-data() -> ()  [unwired: 1 in, 6 out]
      }
    }
    n141 = disable-structure shown="Enabled" {
      disable-tunnel: w63 -> [w71 w73]
      disable-tunnel: [w70 w73] -> w61
      disable-tunnel: [w69 w72] -> w60
      disable-tunnel: w58 -> [_ w72]
      disable-tunnel: [w69 w72] -> w57
      frame Disabled {
        n142 = property on="Table Control" class="Tbl (strict)"(error in=w71) -> (error out=w70:errorcluster, "EditPos"=w69:T2)  [unwired: 1 in, 1 out]
      }
      frame Enabled {
      }
    }
    "Edit Position\n(loop end)" <- w57
    n143 = case shown="True" w65 {
      tunnel: w66 -> [_ w74]
      frame False {
      }
      frame True {
        n144 = local write "Table Control"(w74) -> ()
      }
    }
    "Edit Position\n(loop st)" <- w59
  }
  n145 = local write "Table Control"(w12) -> ()
